vi "Init.vi"(8 "error in (no error)":errorcluster, 9 "y":dbl[](array[numeric]), 10 "x":dbl[](array[numeric]), 11 "Diamond in":refnum<class "Diamond.lvclass">) -> (0 "error out":errorcluster, 3 "Diamond out":refnum<class "Diamond.lvclass">)   [LabVIEW 2021, in "d15.lvlib" / "Diamond.lvclass"]
uses:
  Diamond.lvclass
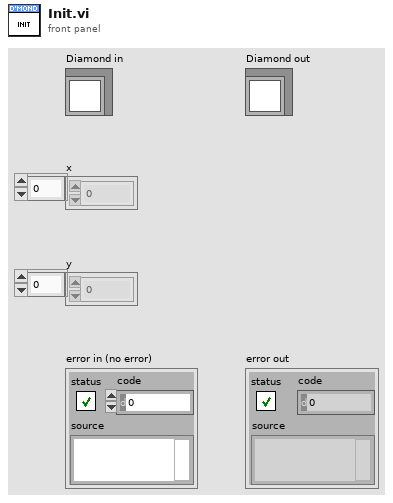
[diagram p1: front panel]
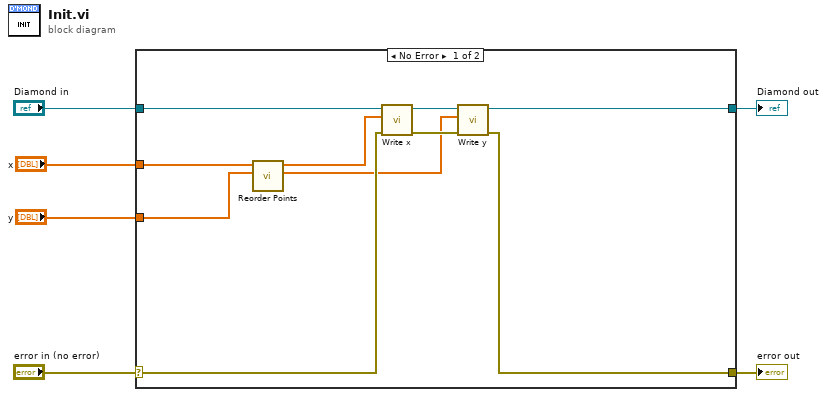
[diagram p0: block diagram]
diagram:
  n1 = case shown="No Error" "error in (no error)" {
    selector: "error in (no error)" -> [w12 w18]
    tunnel: [w11 w18] -> w5
    tunnel: [w14 w17] -> w3
    tunnel: "Diamond in" -> [w16 w17]
    tunnel: "x" -> [w9 _]
    tunnel: "y" -> [w7 _]
    frame No Error {
      n2 = call "Reorder Points.vi"("Y"=w7, "X"=w9) -> ("Y'"=w8:dbl[], "X'"=w10:dbl[])  [unwired: 8 in]
      n3 = call-dynamic "Write x.vi"("error in (no error)"=w12, "x"=w10, "Diamond in"=w16) -> ("error out"=w13:errorcluster, "Diamond out"=w15:refnum<class "Diamond.lvclass">)  [unwired: 7 in]
      n4 = call-dynamic "Write y.vi"("error in (no error)"=w13, "y"=w8, "Diamond in"=w15) -> ("error out"=w11:errorcluster, "Diamond out"=w14:refnum<class "Diamond.lvclass">)  [unwired: 7 in]
    }
    frame Error {
    }
  }
  "error out" <- w5
  "Diamond out" <- w3
